vi "Set-Point Flat-line Signal.vi"(1 "Flatline Offset":dbl format="%0.2p") -> (0 "Flatline Signal":waveform(dbl))   [LabVIEW 2013]
uses:
  <vilib>/measure/NI_MABase.lvlib
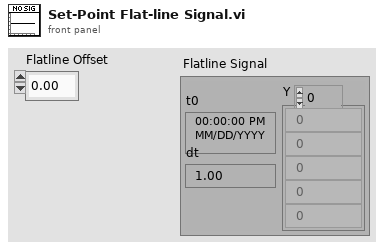
[diagram p1: front panel]
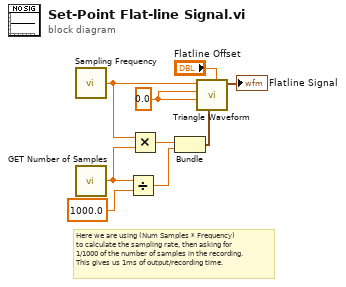
[diagram p0: block diagram]
diagram:
  w6 = 0.0 ("amplitude")
  # "Here we are using (Num Samples * Frequency)\nto calculate the sampling rate, then asking for\n1/1000 of the number of samples in the recording.\nThis gives us 1ms of output/recording time."
  n1 = call "Sampling Frequency.vi"() -> ("Sampling Frequency"=w9:dbl)
  n2 = call "GET Number of Samples.vi"() -> ("Number of Samples"=w3:dbl)
  n3 = Divide(x=w3, y=1000.0) -> (x/y=w2:dbl)
  n4 = Multiply(x=w9, y=w3) -> (x*y=w7:dbl)
  n5 = Bundle(w7, w2) -> (w8:cluster{dbl, dbl})  [unwired: 1 in]
  n6 = call <vilib>:"Triangle Waveform.vi"("offset"="Flatline Offset", "sampling info"=w8, "phase"=w6, "amplitude"=w6, "frequency"=w9) -> ("signal out"=→"Flatline Signal":waveform(dbl))  [unwired: 5 in, 1 out]
